vi "Durability Test Conditions Grabber.vi"(11 "file path":path) -> (3 "Durability Test Conditions":T1)   [LabVIEW 2026]
uses:
  controls/Durability Test Conditions.ctl
  <vilib>/Utility/file.llb/Read Delimited Spreadsheet (string).vi
panel:
  in  "Durability Test Conditions":T1
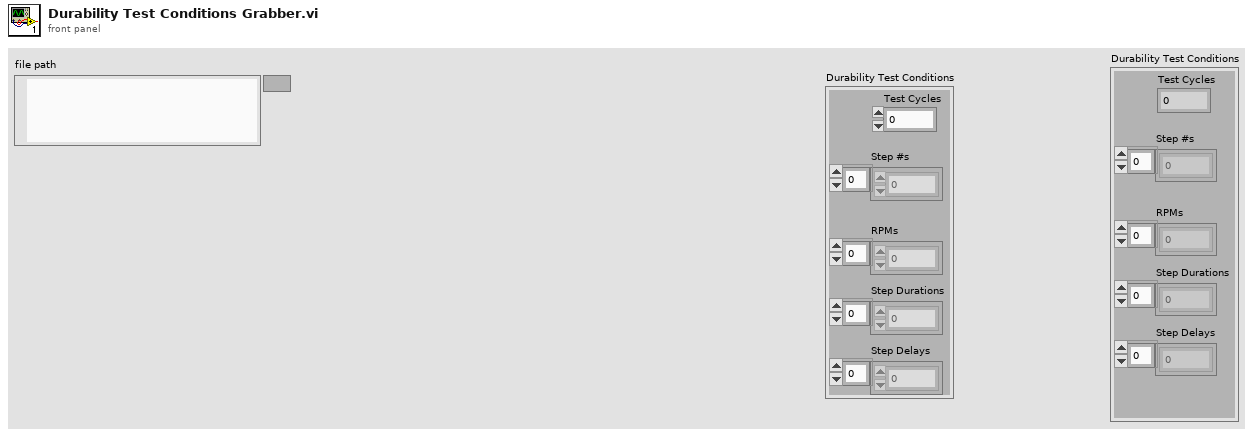
[diagram p1: front panel]
types:
  T1 = typedef "Durability Test Conditions.ctl" = cluster{"Step #s":dbl[], "RPMs":dbl[], "Step Durations":dbl[], "Step Delays":dbl[], "Test Cycles":dbl}
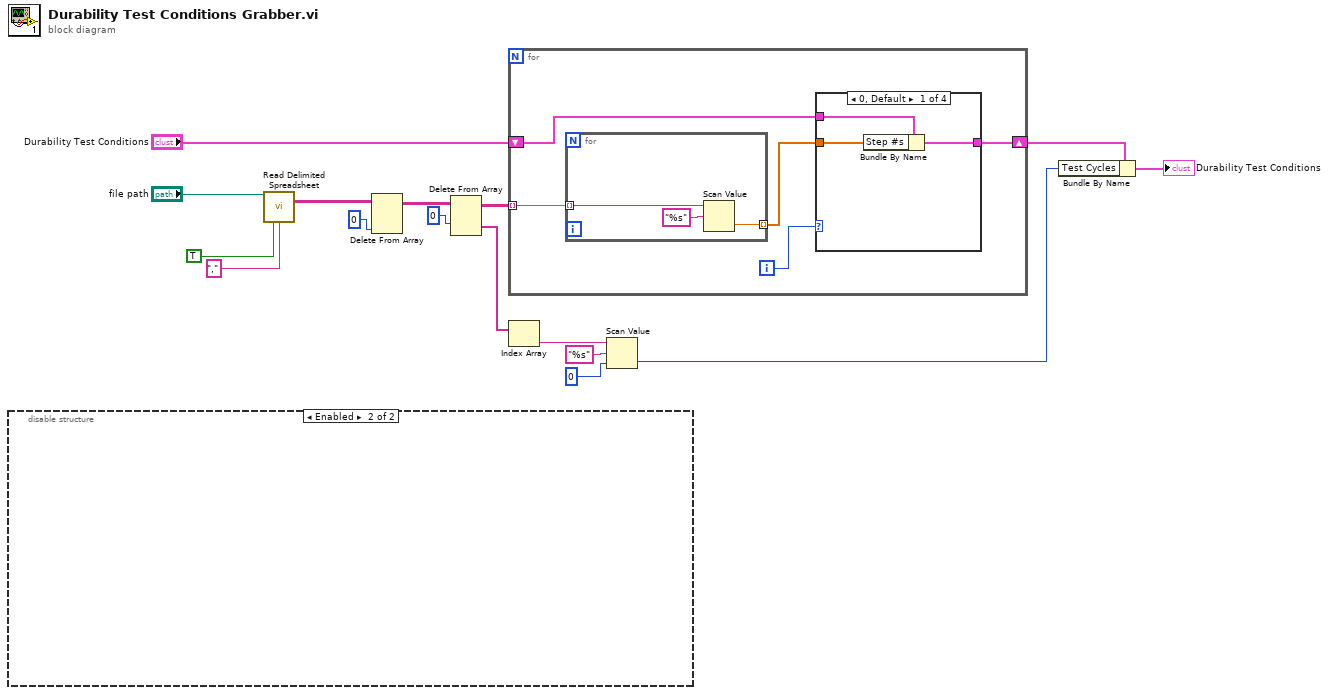
[diagram p0: block diagram]
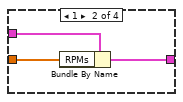
[diagram p2: hidden frame]
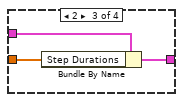
[diagram p3: hidden frame]
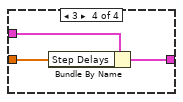
[diagram p4: hidden frame]
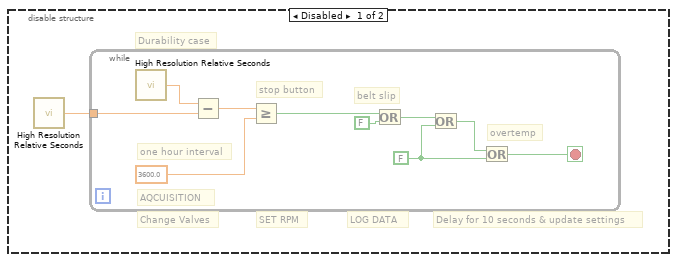
[diagram p5: hidden frame]
diagram:
  n1 = disable-structure shown="Enabled" {
    frame Disabled {
      # "Delay for 10 seconds & update settings"
      # "Change Valves"
      # "Durability case"
      # "LOG DATA"
      # "SET RPM"
      n2 = call <vilib>:"High Resolution Relative Seconds.vi"() -> ("relative seconds"=w17:dbl)
      n3 = while {
        tunnel: w17 -> [w26]
        stop <- w19 stop-if-true
        w18 = FALSE ("y")
        # "one hour interval"
        # "overtemp"
        # "AQCUISITION"
        # "stop button"
        # "belt slip"
        n4 = call <vilib>:"High Resolution Relative Seconds.vi"() -> ("relative seconds"=w27:dbl)
        n5 = Subtract(x=w27, y=w26) -> (x-y=w25:dbl)
        n6 = Greater Or Equal?(x=w25, y=3600.0) -> (x >= y?=w23:bool)
        n7 = Or(x=w23, y=FALSE) -> (x .or. y?=w22:bool)
        n8 = Or(x=w22, y=w18) -> (x .or. y?=w20:bool)
        n9 = Or(x=w20, y=w18) -> (x .or. y?=w19:bool)
      }
    }
    frame Enabled {
    }
  }
  n10 = call-poly <vilib>:"Read Delimited Spreadsheet.vi"("file path (dialog if empty)"="file path", "transpose? (F)"=TRUE, "delimiter (\\t)"="," ("delimiter (\\t)")) -> ("all rows"=w13:string[][])  [unwired: 7 in, 5 out]
  n11 = Delete From Array(array=w13, index (col)=0 ("disabled index (col)")) -> (array with subset deleted=w9:string[][])  [unwired: 2 in, 1 out]
  n12 = Delete From Array(array=w9, index (row)=0) -> (deleted portion=w10:string[], array with subset deleted=w4:string[][])  [unwired: 2 in]
  n13 = for {
    tunnel: w4 -> [w32] mode=indexing
    shift-right: [w29] -> w2
    shift-left: "Durability Test Conditions" -> [w28]
    i -> [w31]
    n14 = for {
      tunnel: w32 -> [w46] mode=indexing
      tunnel: [w45] -> w30 mode=indexing
      n15 = Scan Value(string=w46, format string="%s") -> (value=w45:dbl)  [unwired: 1 in, 1 out]
    }
    n16 = case shown="0, Default" w31 {
      tunnel: w30 -> [w35 w36 w39 w42]
      tunnel: [w34 w37 w40 w43] -> w29
      tunnel: w28 -> [w33 w38 w41 w44]
      frame 0, Default {
        n17 = Bundle By Name(cluster=w33, "Step #s"=w35) -> (w34:T1)
      }
      frame 1 {
        n18 = Bundle By Name(cluster=w38, "RPMs"=w36) -> (w37:T1)
      }
      frame 2 {
        n19 = Bundle By Name(cluster=w41, "Step Durations"=w39) -> (w40:T1)
      }
      frame 3 {
        n20 = Bundle By Name(cluster=w44, "Step Delays"=w42) -> (w43:T1)
      }
    }
  }
  n21 = Index Array(array=w10) -> (element=w8:string)  [unwired: 1 in]
  n22 = Scan Value(string=w8, format string="%s", default (0 dbl)=u16 0) -> (value=w5:u16)  [unwired: 1 out]
  n23 = Bundle By Name(cluster=w2, "Test Cycles"=w5) -> (→"Durability Test Conditions":T1)
